vi "Create Frame Buffer.vi"(8 "error in":errorcluster) -> (0 "error out":errorcluster)   [LabVIEW 2025, in "Automotive Ethernet Bus Monitor.lvclass"]
doc: "Create the frame buffer queue."
uses:
  Automotive Ethernet Bus Monitor.lvclass
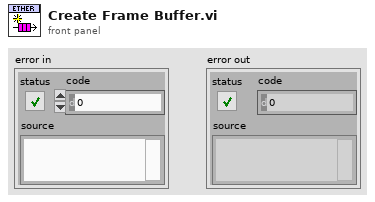
[diagram p1: front panel]
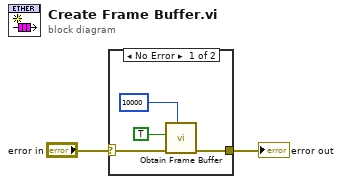
[diagram p0: block diagram]
diagram:
  n1 = case shown="No Error" "error in" {
    selector: "error in" -> [w5 w7]
    tunnel: [w6 w7] -> w1
    frame No Error {
      n2 = call "Obtain Frame Buffer.vi"("Buffer Size (10k)"=10000, "error in"=w5, "Create (F)"=TRUE ("create if not found? (T)")) -> ("error out"=w6:errorcluster)  [unwired: 7 in, 1 out]
    }
    frame Error {
    }
  }
  "error out" <- w1
